vi "Get Image.vi"(7 "Image":T2, 10 "error in (no error)":errorcluster) -> (2 "error out":errorcluster, 3 "Flattened Image":T1)   [LabVIEW 2020, in "TSnax UI.lvlib" / "TSnax UI Manager.lvclass"]
uses:
  TSnax UI Manager.lvclass
  TSnax UI Manager.lvclass/TSnax UI Manager.ctl
  TSnax UI.lvlib
  Image.ctl
  <vilib>/picture/picture.llb/imagedata.ctl
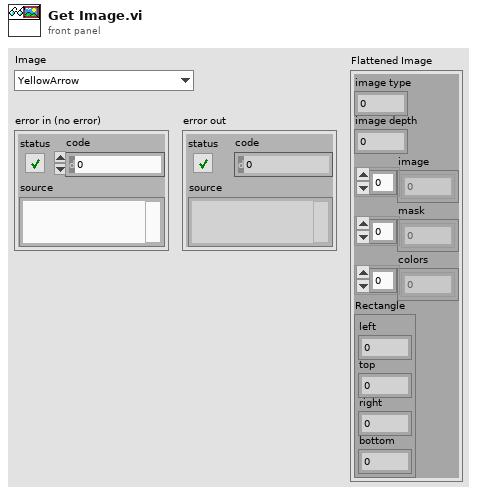
[diagram p1: front panel]
types:
  T1 = typedef "imagedata.ctl" = cluster{"image type":i32, "image depth":i32, "image":u8[], "mask":u8[], "colors":u32[], "Rectangle":cluster{"left":i16, "top":i16, "right":i16, "bottom":i16}}
  T2 = typedef "TSnax UI.lvlib/Image.ctl" = enum16{"YellowArrow", "GreenArrow"}
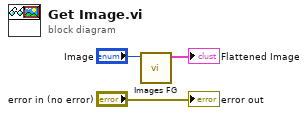
[diagram p0: block diagram]
diagram:
  n1 = call "Images FG.vi"("Image"="Image") -> ("Flattened Image"=→"Flattened Image":T1)  [unwired: 10 in]
  "error out" <- "error in (no error)"
